vi "daemon.vi"(8 "quit":refnum<user-event>, 9 "dvr":refnum<data-value>, 10 "subpanel":refnum<vi>, 11 "mclb":refnum<vi>) -> ()   [LabVIEW 2017, in "rywindow.lvclass"]
uses:
  rywindow.lvclass
  data.ctl
  thread.ctl
  <vilib>/Utility/miscctls.llb/LVFontTypeDef.ctl
  <vilib>/Utility/miscctls.llb/LVPoint32TypeDef.ctl
  rywindow.lvclass/rywindow.ctl
panel:
  out "Drag Mode":enum32{"copy or move", "copy only", "move only"}(ring)
  out "Data":T1(array[cluster])
  out "PlatMods":T2
  out "Mods":cluster{"Double Click":bool, "Menu Key":bool}
  out "Button":u16
  out "Coords":T3
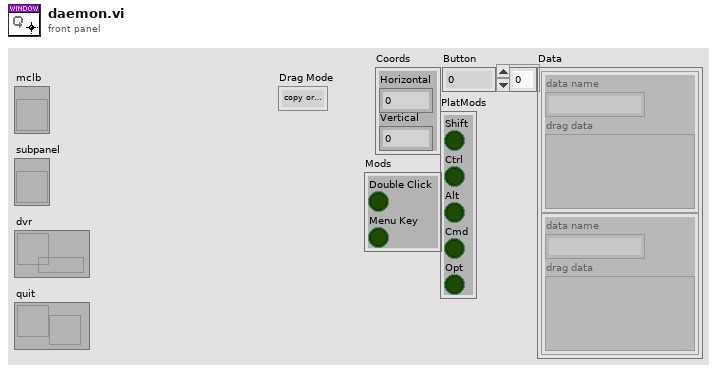
[diagram p1: front panel]
types:
  T1 = cluster{"data name":string, "drag data":variant}[]
  T2 = cluster{"Shift":bool, "Ctrl":bool, "Alt":bool, "Cmd":bool, "Opt":bool}
  T3 = typedef "LVPoint32TypeDef.ctl" = cluster{"Horizontal":i32, "Vertical":i32}
  T4 = typedef "lveventtype.ctl" = enum32{"Null", "Timeout", "Annotation Menu Selection", "Annotation Menu Selection?", "App Instance Close", "App Instance Close?", "Autoscale Range Change", "Bookmark Info Change", "Cell Edit", "Cell Edit?", "Cursor Grab", "Cursor Grab?", "Cursor Menu Selection", "Cursor Menu Selection?", "Cursor Move", "Cursor Release", "Data Change", "Direction Change", "Display State Change", "Drag Ended", "Drag Enter", "Drag Leave", "Drag Over", "Drag Source Update", "Drag Starting", "Drag Starting?", "Drop", "Exec State Change", "Key Down", "Key Down?", "Key Repeat", "Key Repeat?", "Key Up", "Listbox Double Click", "Menu Activation?", "Menu Selection (App)", "Menu Selection? (App)", "Menu Selection (User)", "Mouse Down", "Mouse Down?", "Mouse Enter", "Mouse Leave", "Mouse Move", "Mouse Up", "Mouse Wheel", "NI Security User Change (App)", "Pane Size", "Panel Close", "Panel Close?", "Panel Resize", "Plot Attribute Change", "Scale Range Change", "Shortcut Menu Activation?", "Shortcut Menu Selection (App)", "Shortcut Menu Selection? (App)", "Shortcut Menu Selection (User)", "Tree Double Click", "Tree Drag", "Tree Drag?", "Tree Drop", "Tree Drop?", "Tree Item Close", "Tree Item Close?", "Tree Item Open", "Tree Item Open?", "User Event", "Value Change"}
  T5 = typedef "LVRectTypeDef.ctl" = cluster{"Left":i16, "Top":i16, "Right":i16, "Bottom":i16}
  T6 = typedef "sizeaction.ctl" = enum32{"Minimized", "Maximized", "Resized"}
  T7 = typedef "panelstate.ctl" = enum32{"Standard", "Minimized", "Maximized"}
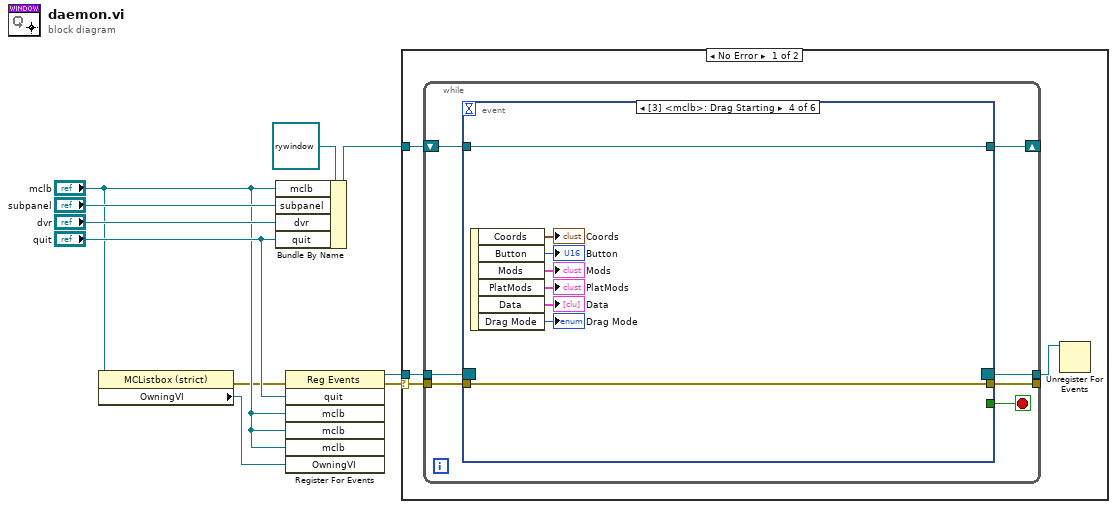
[diagram p0: block diagram]
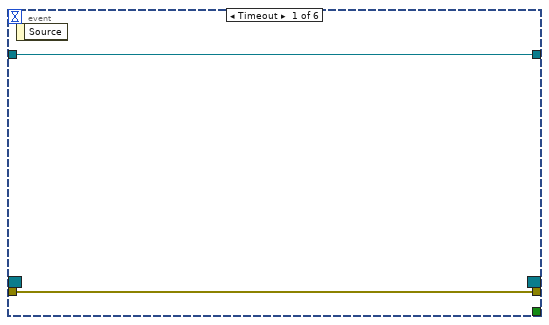
[diagram p2: hidden frame]
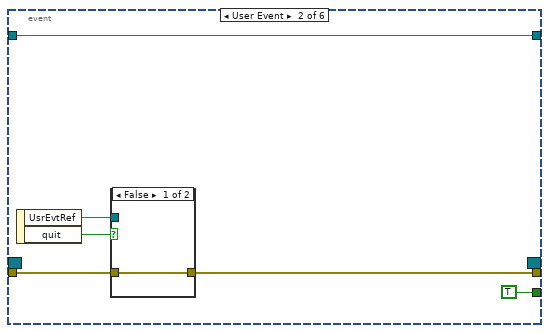
[diagram p3: hidden frame]
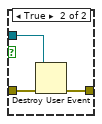
[diagram p4: hidden frame]
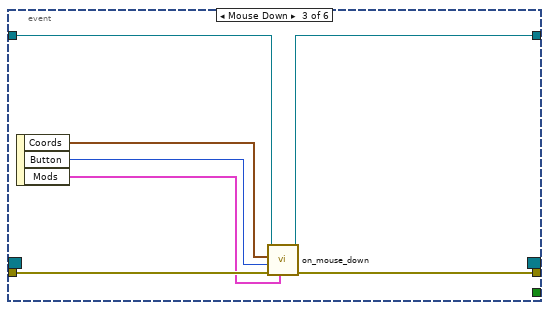
[diagram p5: hidden frame]
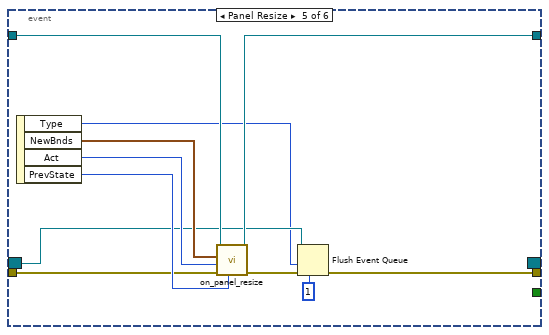
[diagram p6: hidden frame]
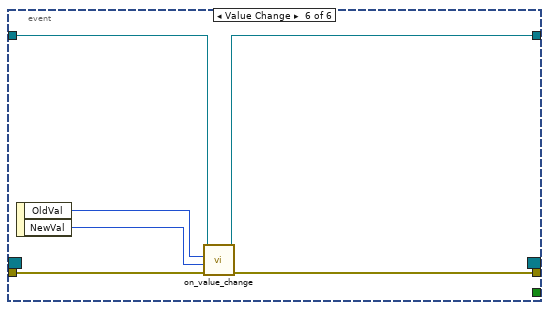
[diagram p7: hidden frame]
diagram:
  n1 = property class="MCListbox (strict)"(reference="mclb") -> (error out=w2:errorcluster, "OwningVI"=w1:refnum<vi>)  [unwired: 1 in, 1 out]
  n2 = Bundle By Name(cluster=refnum<class "rywindow.lvclass"> refnum ("window"), "mclb"="mclb", "subpanel"="subpanel", "dvr"="dvr", "quit"="quit") -> (w4:refnum<class "rywindow.lvclass">)
  n3 = register-events(error in=w2, "quit", "mclb", "mclb", "mclb", w1) -> (reference out=w5:refnum<event-registration>, error out=w6:errorcluster)  [unwired: 1 in]
  n4 = case shown="No Error" w6 {
    selector: w6 -> [w14 _]
    tunnel: w5 -> [w13 _]
    tunnel: w4 -> [w11 _]
    frame No Error {
      n5 = while {
        tunnel: w14 -> [w21]
        tunnel: w13 -> [w20]
        tunnel: [w19] -> _
        tunnel: [w18] -> w12
        shift-right: [w16] -> _
        shift-left: w11 -> [w15]
        stop <- w17 stop-if-true
        n6 = event shown="[3] <mclb>: Drag Starting" {
          selector: w20 -> [_ _ _ _ w54 _]
          dyn-events: [_ _ _ _ _ _] -> w18
          timeout: _ -> [_ _ _ _ _ _]
          tunnel: w21 -> [w23 w29 w40 w48 w51 w65]
          tunnel: [w23 w28 w39 w48 w50 w64] -> w19
          tunnel: [_ TRUE _ _ _ _] -> w17
          tunnel: [w22 w24 w37 w47 w58 w62] -> w16
          tunnel: w15 -> [w22 w24 w38 w47 w59 w63]
          event Timeout {
            n7 = event-data() -> ()  [unwired: 1 in, 1 out]
          }
          event User Event {
            n8 = event-data() -> ("UsrEvtRef"=w27:refnum<user-event>, "quit"=w26:bool)  [unwired: 1 in]
            n9 = case shown="False" w26 {
              tunnel: w29 -> [w30 w33]
              tunnel: [w30 w32] -> w28
              tunnel: w27 -> [_ w31]
              frame False {
              }
              frame True {
                n10 = Destroy User Event(user event=w31, error in=w33) -> (error out=w32:errorcluster)
              }
            }
          }
          event Mouse Down {
            n11 = event-data() -> ("Coords"=w36:T3, "Button"=w35:u16, "Mods"=w34:cluster{"Double Click":bool, "Menu Key":bool})  [unwired: 1 in]
            n12 = call "on_mouse_down.vi"("Mods"=w34, "error in (no error)"=w40, "Button"=w35, "Coords"=w36, "window in"=w38) -> ("error out"=w39:errorcluster, "window out"=w37:refnum<class "rywindow.lvclass">)  [unwired: 5 in]
          }
          event Drag Starting {
            n13 = event-data() -> ("Coords"=→"Coords":T3, "Button"=→"Button":u16, "Mods"=→"Mods":cluster{"Double Click":bool, "Menu Key":bool}, "PlatMods"=→"PlatMods":T2, "Data"=→"Data":T1, "Drag Mode"=→"Drag Mode":enum32{"copy or move", "copy only", "move only"})  [unwired: 1 in]
          }
          event Panel Resize {
            n14 = event-data() -> ("Type"=w49:T4, "NewBnds"=w57:T5, "Act"=w56:T6, "PrevState"=w55:T7)  [unwired: 1 in]
            n15 = call "on_panel_resize.vi"("PrevState"=w55, "error in (no error)"=w51, "Act"=w56, "NewBnds"=w57, "window in"=w59) -> ("error out"=w52:errorcluster, "window out"=w58:refnum<class "rywindow.lvclass">)  [unwired: 5 in]
            n16 = Flush Event Queue(0:w54, 2:w49, 3:w52, 5:1 ("keep most recent")) -> (11:w50:errorcluster)  [unwired: 2 in, 2 out]
          }
          event Value Change {
            n17 = event-data() -> ("OldVal"=w61:i32, "NewVal"=w60:i32)  [unwired: 1 in]
            n18 = call "on_value_change.vi"("error in (no error)"=w65, "NewVal"=w60, "OldVal"=w61, "window in"=w63) -> ("error out"=w64:errorcluster, "window out"=w62:refnum<class "rywindow.lvclass">)  [unwired: 6 in]
          }
        }
      }
      n19 = Unregister For Events(event registration refnum=w12) -> ()  [unwired: 1 in, 1 out]
    }
    frame Error {
    }
  }
